vi "getRef.vi"(5 "error in (no error)":errorcluster) -> (16 "check_in_ref":refnum<class "checkIN.lvclass">, 19 "error out":errorcluster)   [LabVIEW 2015, in "checkIN.lvclass"]
uses:
  checkIN.lvclass
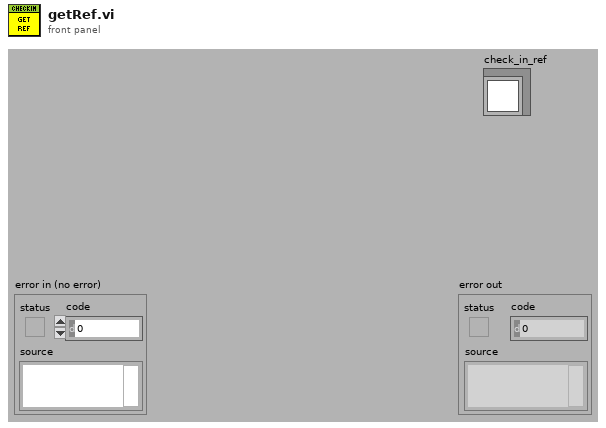
[diagram p1: front panel]
types:
  T1 = typedef "checkIN.lvclass/ClassAttributesRef.ctl" = refnum<data-value>
  T2 = typedef "checkIN.lvclass/ClassAttributes.ctl" = cluster{"Dummy":bool, "check_in_refs":refnum<class "checkIN.lvclass">[]}
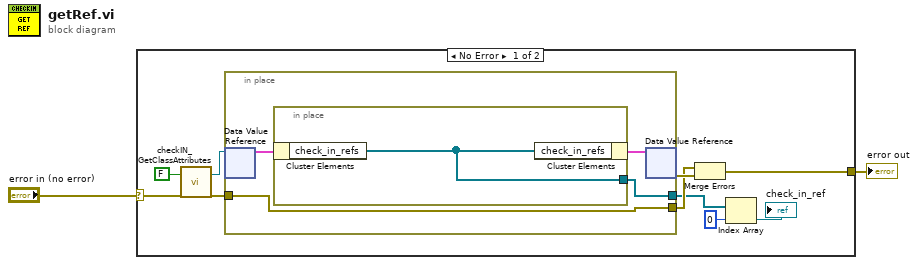
[diagram p0: block diagram]
diagram:
  n1 = case shown="No Error" "error in (no error)" {
    selector: "error in (no error)" -> [w8 w18]
    tunnel: [w12 w18] -> w1
    frame No Error {
      n2 = call "checkIN_GetClassAttributes.vi"("return data? (T)"=FALSE, "error in (no error)"=w8) -> ("class attributes ref"=w6:T1, "error out"=w7:errorcluster)  [unwired: 14 in, 2 out]
      n3 = in-place {
        in-place-border: w7 -> [w14]
        in-place-border: [w14] -> w10
        in-place-border: [w13] -> w5
        n4 = in-place-dvr #1(w6) -> (w15:T2)  [unwired: 1 out]
        n5 = in-place {
          in-place-border: [w17] -> w13
          n6 = in-place-cluster #2(w15) -> ("check_in_refs"=w17:refnum<class "checkIN.lvclass">[])
          n7 = in-place-cluster #2("check_in_refs"=w17) -> (w16:T2)
        }
        n8 = in-place-dvr #1(w16) -> (w11:errorcluster)  [unwired: 1 out]
      }
      n9 = Merge Errors(w10, w11) -> (w12:errorcluster)
      n10 = Index Array(array=w5, index=0) -> (element=→"check_in_ref":refnum<class "checkIN.lvclass">)
    }
    frame Error {
    }
  }
  "error out" <- w1
